vi "SV Close File.vi"(0 "file refnum":refnum<file>, 11 "error in":errorcluster) -> (4 "file path":path, 15 "error out":errorcluster)   [LabVIEW 2017, in "SoundVib_UFF58.lvlib"]
doc: "Closes the UFF58 (universal file format) file specified by <B>file refnum</B>."
uses:
  <vilib>/addons/Sound and Vibration/svt_UFF58/SoundVib_UFF58.lvlib
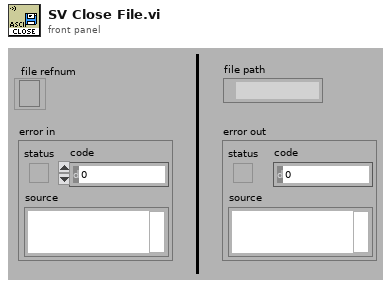
[diagram p1: front panel]
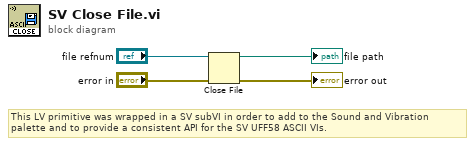
[diagram p0: block diagram]
diagram:
  # "This LV primitive was wrapped in a SV subVI in order to add to the Sound and Vibration palette and to provide a consistent API for the SV UFF58 ASCII VIs."
  n1 = Close File(refnum="file refnum", error in="error in") -> (path=→"file path":path, error out=→"error out":errorcluster)
